vi "Station_Wise_Enable_Disable_Main_Indi.vi"(8 "error in (no error)":errorcluster, 9 "Station number":string[](array[string]), 10 "Station name":string[](array[string]), 11 "appended array":refnum<vi>[](array[refnum])) -> (0 "error out":errorcluster, 3 "Valid Indicators":refnum<vi>[](array[refnum]))   [LabVIEW 2017]
doc: "This vi is used to diable the main indicators in Station_Wise_VI AND this vi is used to name the indicator with station names"
panel:
  in  "Station 7":bool
  out "Display 1":T1
  # "Communication:-"
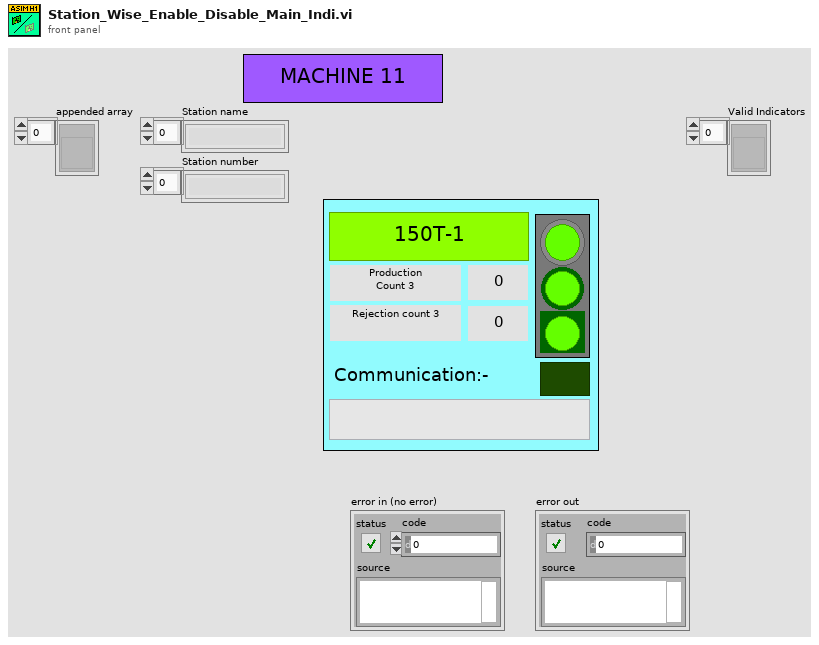
[diagram p1: front panel]
types:
  T1 = cluster{"Status 10":cluster{"S":bool, "l":bool, "M":bool, "Q":bool, "P":bool}, "Station Name":bool, "Production\nCount 3":i32, "Rejection count 3":i32, "String Indicator 3":bool, "Product code 10":string}
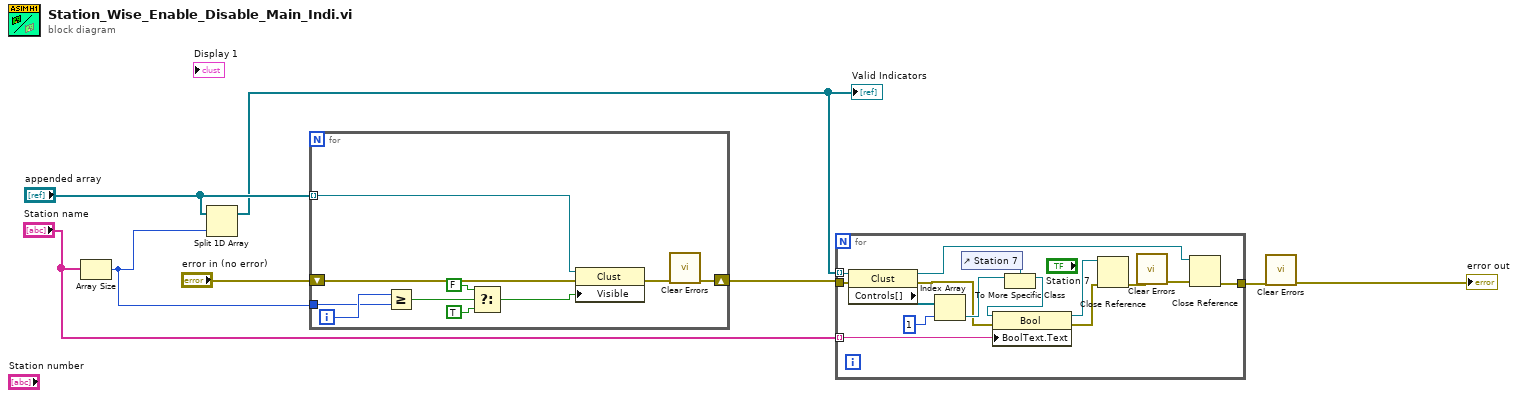
[diagram p0: block diagram]
diagram:
  n1 = Array Size(array="Station name") -> (size(s)=w6:i32)
  n2 = Split 1D Array(array="appended array", index=w6) -> (first subarray=w5:refnum<vi>[])  [unwired: 1 out]
  "Valid Indicators" <- w5
  n3 = for {
    shift-right: [w16] -> w4
    shift-left: "error in (no error)" -> [w18]
    tunnel: "appended array" -> [w9] mode=indexing
    tunnel: w6 -> [w14]
    i -> [w15]
    n4 = Greater Or Equal?(x=w15, y=w14) -> (x >= y?=w13:bool)
    n5 = Select(t=FALSE, s=w13, f=TRUE) -> (s? t:f=w10:bool)
    n6 = property on="Property Node" class="Clust"(reference=w9, error in=w18, "Visible"=w10) -> (error out=w17:errorcluster)  [unwired: 1 out]
    n7 = call <vilib>:"Clear Errors.vi"("error in (no error)"=w17) -> ("error out"=w16:errorcluster)  [unwired: 5 in, 1 out]
  }
  n8 = for {
    tunnel: "Station name" -> [w28] mode=indexing
    tunnel: w5 -> [w27] mode=indexing
    tunnel: w4 -> [w26]
    tunnel: [w21] -> w1
    n9 = property on="Property Node" class="Clust"(reference=w27, error in=w26) -> (reference out=w22:refnum<vi>, error out=w25:errorcluster, "Controls[]"=w33:refnum<vi>[])
    n10 = Index Array(array=w33, index=1) -> (element=w31:refnum<vi>)
    n11 = control-ref of="Station 7"() -> (w30:refnum<vi>)
    n12 = To More Specific Class(target class=w30, reference=w31) -> (specific class reference=w29:refnum<vi>)  [unwired: 1 in, 1 out]
    n13 = property on="Property Node" class="Bool"(reference=w29, error in=w25, "BoolText.Text"=w28) -> (reference out=w24:refnum<vi>, error out=w23:errorcluster)
    n14 = Close Reference(reference=w24, error in (no error)=w23) -> (error out=w20:errorcluster)
    n15 = call <vilib>:"Clear Errors.vi"("error in (no error)"=w20) -> ("error out"=w19:errorcluster)  [unwired: 5 in, 1 out]
    n16 = Close Reference(reference=w22, error in (no error)=w19) -> (error out=w21:errorcluster)
  }
  n17 = call <vilib>:"Clear Errors.vi"("error in (no error)"=w1) -> ("error out"=→"error out":errorcluster)  [unwired: 5 in, 1 out]
